vi "DHE_Aliases.vi"(5 "expand reg":bool, 7 "action":T2(ring)=enum."find", 10 "name in":string) -> (1 "found?":bool, 2 "name out":string, 3 "aliases":T1[](array[typedef]), 4 "register?":bool)   [LabVIEW 2016]
uses:
  private/vis/DHE_alias.ctl
  <vilib>/Utility/config.llb/Read Key (String).vi
  <vilib>/Utility/config.llb/NI_LVConfig.lvlib
panel:
  in  "alias":T1
  in  "error in (no error)":errorcluster
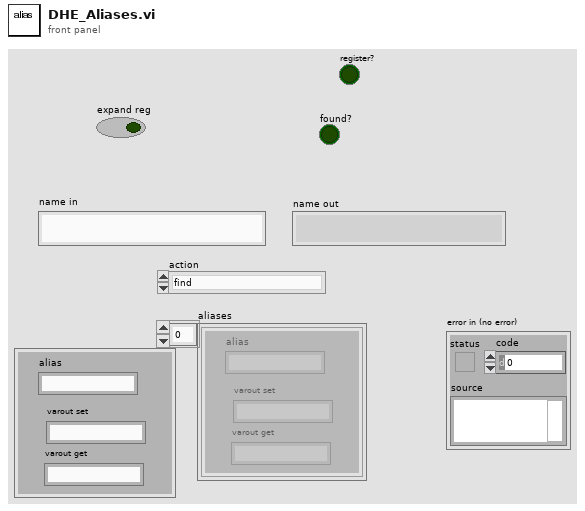
[diagram p1: front panel]
types:
  T1 = typedef "DHE_alias.ctl" = cluster{"alias":string, "varout set":string, "varout get":string}
  T2 = enum16{"read from file", "find", "get", "add", "delete", "clear "}
  T3 = typedef "NI_LVConfig.lvlib/Config Data RefNum.ctl" = refnum<k1>
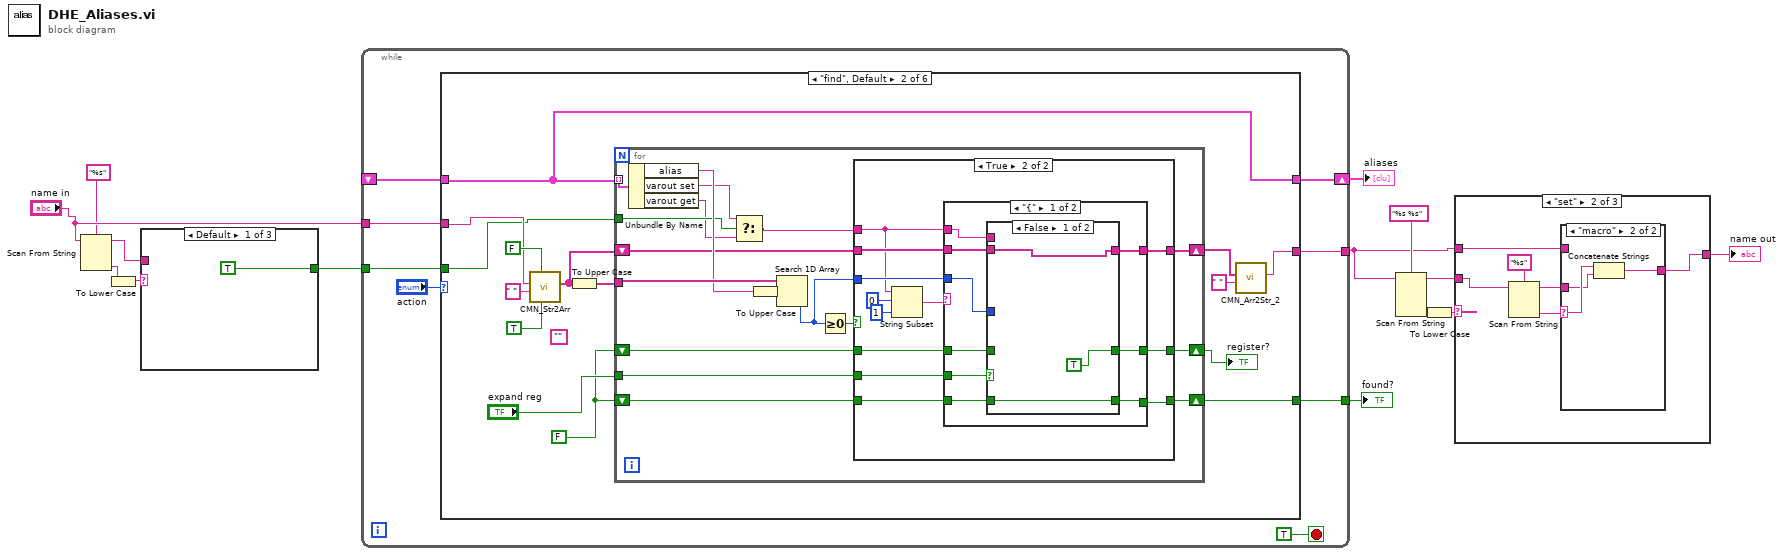
[diagram p0: block diagram]
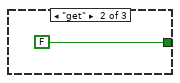
[diagram p2: hidden frame]
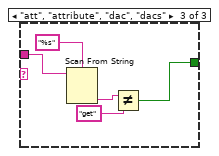
[diagram p3: hidden frame]
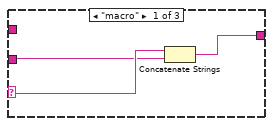
[diagram p4: hidden frame]
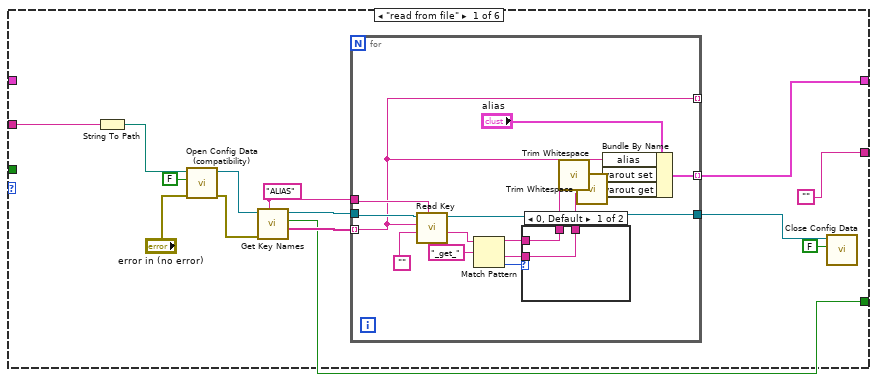
[diagram p7: hidden frame]
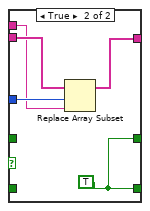
[diagram p10: hidden frame]
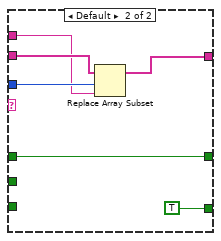
[diagram p11: hidden frame]
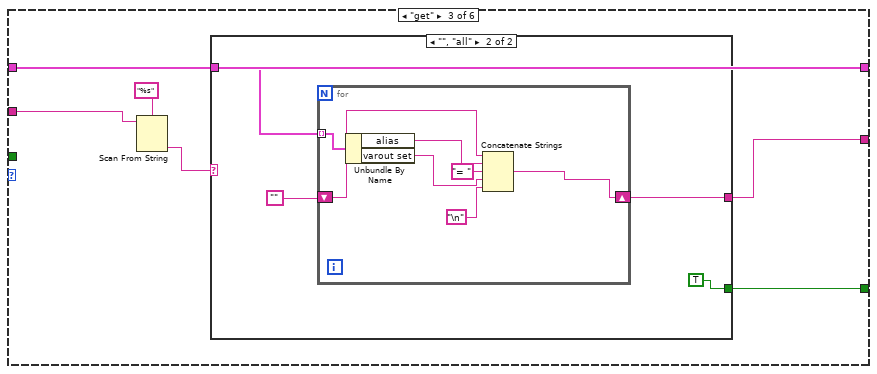
[diagram p12: hidden frame]
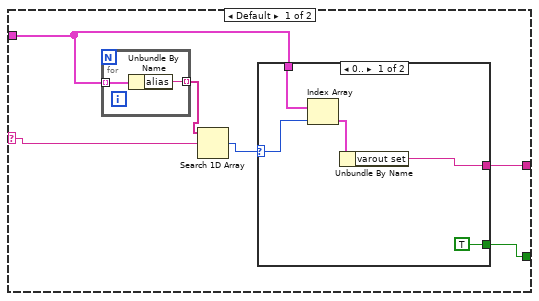
[diagram p13: hidden frame]
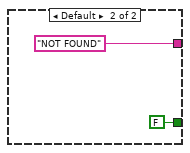
[diagram p14: hidden frame]
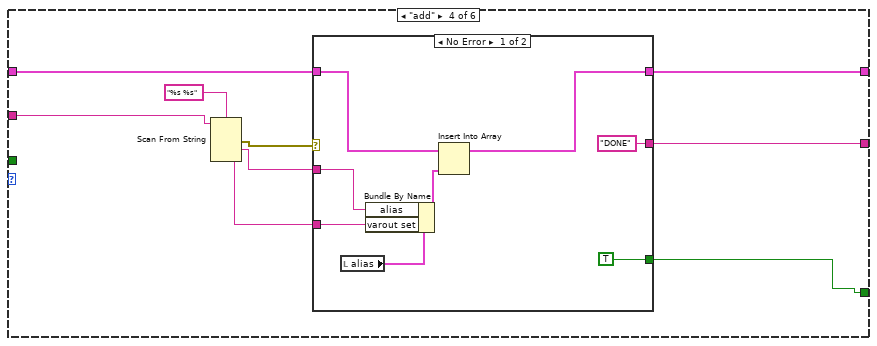
[diagram p15: hidden frame]
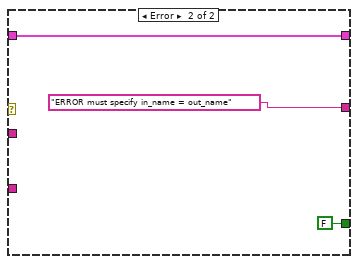
[diagram p16: hidden frame]
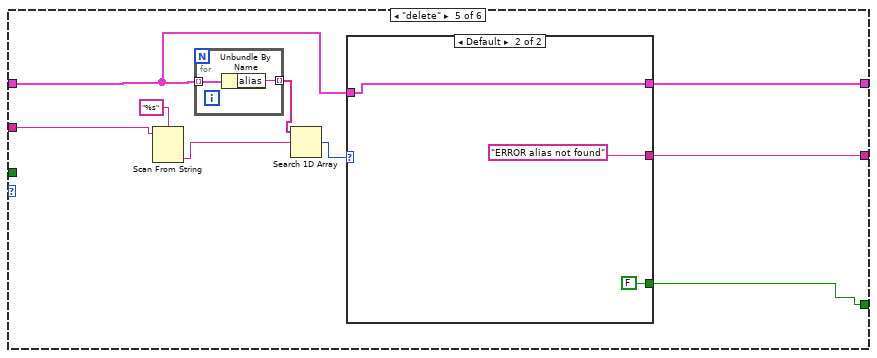
[diagram p17: hidden frame]
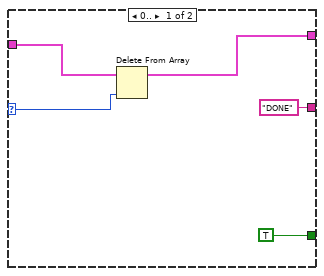
[diagram p18: hidden frame]
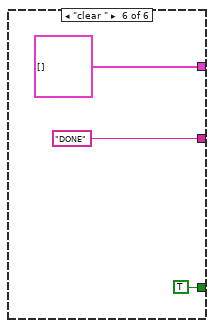
[diagram p19: hidden frame]
diagram:
  n1 = Scan From String(format string="%s", input string="name in") -> (remaining string=w2:string, output 1=w4:string)  [unwired: 3 in, 2 out]
  n2 = To Lower Case(string=w4) -> (all lower case string=w3:string)
  n3 = case shown="Default" w3 {
    tunnel: [TRUE FALSE w17] -> w1
    tunnel: w2 -> [_ _ w21]
    frame Default {
    }
    frame "get" {
    }
    frame "att", "attribute", "dac", "dacs" {
      n4 = Scan From String(format string="%s", input string=w21) -> (output 1=w19:string)  [unwired: 3 in, 3 out]
      n5 = Not Equal?(x=w19, y="get") -> (x != y?=w17:bool)
    }
  }
  n6 = while {
    shift-right: [w28] -> w14
    shift-left: _ -> [w27]
    tunnel: [w25] -> w8
    tunnel: [w24] -> w13
    tunnel: "name in" -> [w23]
    tunnel: w1 -> [w22]
    stop <- TRUE stop-if-true
    n7 = case shown="\"find\", Default" "action" {
      tunnel: [w37 w77 w138 w167 w191 T1[] []] -> w28
      tunnel: w27 -> [_ w77 w138 w173 w186 _]
      tunnel: w23 -> [w35 w64 w136 w172 w193 _]
      tunnel: ["" w70 w137 w166 w190 "DONE" ("string out")] -> w25
      tunnel: [w30 w68 w133 w165 w185 TRUE ("section exists?")] -> w24
      tunnel: w22 -> [_ w63 _ _ _ _]
      frame "read from file" {
        w43 = "ALIAS" ("section")
        n8 = String To Path(string=w35) -> (path=w34:path)
        n9 = call <vilib>:"Open Config Data (compatibility).vi"("error in (no error)"="error in (no error)", "create file if necessary (T)"=FALSE, "configuration file path"=w34) -> ("error out"=w39:errorcluster, "refnum"=w38:T3)  [unwired: 6 in, 1 out]
        n10 = call <vilib>:"Get Key Names.vi"("section"=w43, "error in (no error)"=w39, "refnum"=w38) -> ("key names"=w42:string[], "section exists?"=w30:bool, "refnum out"=w41:T3)  [unwired: 6 out]
        n11 = for {
          tunnel: w41 -> [w59]
          tunnel: w43 -> [w58]
          tunnel: w42 -> [w54] mode=indexing
          tunnel: [w55] -> w37 mode=indexing
          tunnel: [w54] -> _ mode=indexing
          tunnel: [w53] -> w32
          n12 = call-poly <vilib>:"Read Key.vi"("section"=w58, "default value"="", "key"=w54, "refnum"=w59) -> ("value"=w52:string, "refnum out"=w53:T3)  [unwired: 2 in, 4 out]
          n13 = Match Pattern(string=w52, regular expression="_get_") -> (before substring=w48:string, after substring=w49:string, offset past match=w50:i32)  [unwired: 1 in, 1 out]
          n14 = case shown="0, Default" w50 {
            tunnel: w49 -> [w60 _]
            tunnel: w48 -> [w61 w62]
            tunnel: [w61 w62] -> w47
            tunnel: [w60 w62] -> w46
            frame 0, Default {
            }
            frame ..-1 {
            }
          }
          n15 = call <vilib>:"Trim Whitespace.vi"("string"=w47) -> ("trimmed string"=w45:string)  [unwired: 1 in]
          n16 = call <vilib>:"Trim Whitespace.vi"("string"=w46) -> ("trimmed string"=w44:string)  [unwired: 1 in]
          n17 = Bundle By Name(cluster="alias", "alias"=w54, "varout set"=w45, "varout get"=w44) -> (w55:T1)
        }
        n18 = call <vilib>:"Close Config Data.vi"("write file if changed (T)"=FALSE, "refnum"=w32) -> ()  [unwired: 8 in, 2 out]
      }
      frame "find", Default {
        w67 = FALSE
        (unwired) ""
        n19 = call "CMN_Str2Arr.vi"("trim"=TRUE, "strip quotation marks"=FALSE, "separator"=" ", "string in"=w64) -> ("Array out"=w73:string[])  [unwired: 7 in]
        n20 = To Upper Case(1:w73) -> (0:w65:string[])
        n21 = for {
          tunnel: w77 -> [w94] mode=indexing
          tunnel: w65 -> [w93]
          shift-right: [w88] -> w72
          shift-left: w73 -> [w90]
          tunnel: "expand reg" -> [w87]
          shift-right: [w85] -> w68
          shift-left: w67 -> [w86]
          shift-right: [w83] -> w66
          shift-left: w67 -> [w84]
          tunnel: w63 -> [w81]
          n22 = Unbundle By Name(w94) -> ("alias"=w92:string, "varout set"=w80:string, "varout get"=w79:string)
          n23 = Select(t=w80, s=w81, f=w79) -> (s? t:f=w78:string)
          n24 = To Upper Case(1:w92) -> (0:w82:string)
          n25 = Search 1D Array(1D array=w93, element=w82) -> (index of element=w89:i32)  [unwired: 1 in]
          n26 = Greater Or Equal To 0?(x=w89) -> (x >= 0?=w91:bool)
          n27 = case shown="True" w91 {
            tunnel: w90 -> [w97 w109]
            tunnel: w89 -> [_ w108]
            tunnel: w78 -> [_ w106]
            tunnel: [w97 w107] -> w88
            tunnel: w87 -> [_ w102]
            tunnel: w86 -> [w96 w101]
            tunnel: [w96 w100] -> w85
            tunnel: w84 -> [w95 w99]
            tunnel: [w95 w98] -> w83
            frame False {
            }
            frame True {
              n28 = String Subset(string=w106, offset (0)=0, length (rest)=1 ("length (rest)")) -> (substring=w103:string)
              n29 = case shown="\"{\"" w103 {
                tunnel: w109 -> [w117 w132]
                tunnel: w108 -> [w116 w131]
                tunnel: w106 -> [w115 w130]
                tunnel: [w114 w129] -> w107
                tunnel: w102 -> [w118 _]
                tunnel: w101 -> [w113 _]
                tunnel: [w112 TRUE] -> w100
                tunnel: w99 -> [w111 w127]
                tunnel: [w110 w127] -> w98
                frame "{" {
                  n30 = case shown="False" w118 {
                    tunnel: w117 -> [w121 w125]
                    tunnel: w116 -> [_ w126]
                    tunnel: w115 -> [_ w124]
                    tunnel: [w121 w123] -> w114
                    tunnel: w113 -> [w120 _]
                    tunnel: [w120 w122] -> w112
                    tunnel: w111 -> [_ _]
                    tunnel: [TRUE w122] -> w110
                    frame False {
                    }
                    frame True {
                      w122 = TRUE
                      n31 = Replace Array Subset(array=w125, new element=w124, index=w126) -> (w123:string[])
                    }
                  }
                }
                frame Default {
                  n32 = Replace Array Subset(array=w132, new element=w130, index=w131) -> (w129:string[])
                }
              }
            }
          }
        }
        "register?" <- w66
        n33 = call "CMN_Arr2Str_2.vi"("separator"=" ", "Array in"=w72) -> ("string out"=w70:string)  [unwired: 9 in]
      }
      frame "get" {
        n34 = Scan From String(format string="%s", input string=w136) -> (output 1=w134:string)  [unwired: 3 in, 3 out]
        n35 = case shown="\"\", \"all\"" w134 {
          selector: w134 -> [w143 _]
          tunnel: w138 -> [w141 w157]
          tunnel: [w140 w155] -> w137
          tunnel: [w139 TRUE ("section exists?")] -> w133
          frame Default {
            n36 = for {
              tunnel: w141 -> [w153] mode=indexing
              tunnel: [w152] -> w144 mode=indexing
              n37 = Unbundle By Name(w153) -> ("alias"=w152:string)
            }
            n38 = Search 1D Array(1D array=w144, element=w143) -> (index of element=w142:i32)  [unwired: 1 in]
            n39 = case shown="0.." w142 {
              selector: w142 -> [w148 _]
              tunnel: w141 -> [w149 _]
              tunnel: [w146 "NOT FOUND" ("varout")] -> w140
              tunnel: [TRUE ("section exists?") FALSE ("section exists?")] -> w139
              frame 0.. {
                n40 = Index Array(array=w149, index=w148) -> (element=w147:T1)
                n41 = Unbundle By Name(w147) -> ("varout set"=w146:string)
              }
              frame Default {
              }
            }
          }
          frame "", "all" {
            n42 = for {
              tunnel: w157 -> [w164] mode=indexing
              shift-right: [w158] -> w155
              shift-left: "" -> [w159]
              n43 = Unbundle By Name(w164) -> ("alias"=w163:string, "varout set"=w161:string)
              n44 = Concatenate Strings(w159, w163, "= " ("string"), w161, "\n") -> (w158:string)
            }
          }
        }
      }
      frame "add" {
        n45 = Scan From String(format string="%s %s", input string=w172) -> (error out=w170:errorcluster, output 1=w169:string, output 2=w168:string)  [unwired: 4 in, 2 out]
        n46 = case shown="No Error" w170 {
          tunnel: w173 -> [w181 w184]
          tunnel: w169 -> [w179 _]
          tunnel: w168 -> [w178 _]
          tunnel: [w176 w184] -> w167
          tunnel: ["DONE" ("string out") "ERROR must specify in_name = out_name" ("string out")] -> w166
          tunnel: [TRUE ("section exists?") FALSE ("section exists?")] -> w165
          frame No Error {
            n47 = local read "alias"() -> (w180:T1)
            n48 = Bundle By Name(cluster=w180, "alias"=w179, "varout set"=w178) -> (w177:T1)
            n49 = Insert Into Array(array=w181, new element=w177) -> (w176:T1[])  [unwired: 1 in]
          }
          frame Error {
          }
        }
      }
      frame "delete" {
        n50 = Scan From String(format string="%s", input string=w193) -> (output 1=w188:string)  [unwired: 3 in, 3 out]
        n51 = for {
          tunnel: w186 -> [w195] mode=indexing
          tunnel: [w194] -> w189 mode=indexing
          n52 = Unbundle By Name(w195) -> ("alias"=w194:string)
        }
        n53 = Search 1D Array(1D array=w189, element=w188) -> (index of element=w187:i32)  [unwired: 1 in]
        n54 = case shown="Default" w187 {
          selector: w187 -> [w198 _]
          tunnel: [w197 w202] -> w191
          tunnel: ["DONE" ("string out") "ERROR alias not found" ("string out")] -> w190
          tunnel: w186 -> [w199 w202]
          tunnel: [TRUE ("section exists?") FALSE ("section exists?")] -> w185
          frame 0.. {
            n55 = Delete From Array(array=w199, index=w198) -> (array with subset deleted=w197:T1[])  [unwired: 1 in, 1 out]
          }
          frame Default {
          }
        }
      }
      frame "clear " {
      }
    }
  }
  "aliases" <- w14
  "found?" <- w13
  n56 = Scan From String(format string="%s %s", input string=w8) -> (remaining string=w10:string, output 2=w11:string)  [unwired: 5 in, 2 out]
  n57 = To Lower Case(string=w11) -> (all lower case string=w9:string)
  n58 = case shown="\"set\"" w9 {
    selector: w9 -> [w209 _ _]
    tunnel: w10 -> [w208 w215 _]
    tunnel: w8 -> [_ w210 w220]
    tunnel: [w207 w211 w220] -> w7
    frame "macro" {
      n59 = Concatenate Strings(w209, w208) -> (w207:string)
    }
    frame "set" {
      n60 = Scan From String(format string="%s", input string=w215) -> (remaining string=w212:string, output 1=w213:string)  [unwired: 3 in, 2 out]
      n61 = case shown="\"macro\"" w213 {
        selector: w213 -> [_ w219]
        tunnel: w212 -> [_ w218]
        tunnel: [w216 w217] -> w211
        tunnel: w210 -> [w216 _]
        frame Default {
        }
        frame "macro" {
          n62 = Concatenate Strings(w219, w218) -> (w217:string)
        }
      }
    }
    frame Default {
    }
  }
  "name out" <- w7
